vi "Plot menu activation.vi"(8 "error in (no error)":errorcluster, 11 "BluePlotHandle in":refnum<class "BluePlotHandle.lvclass">) -> (0 "error out":errorcluster, 2 "item tags":string[](array[string]), 3 "BluePlotHandle out":refnum<class "BluePlotHandle.lvclass">)   [LabVIEW 2021, in "BluePlot.lvlib" / "BluePlotHandle.lvclass"]
uses:
  BluePlotHandle.lvclass
  BluePlotHandle.lvclass/BluePlotHandle.ctl
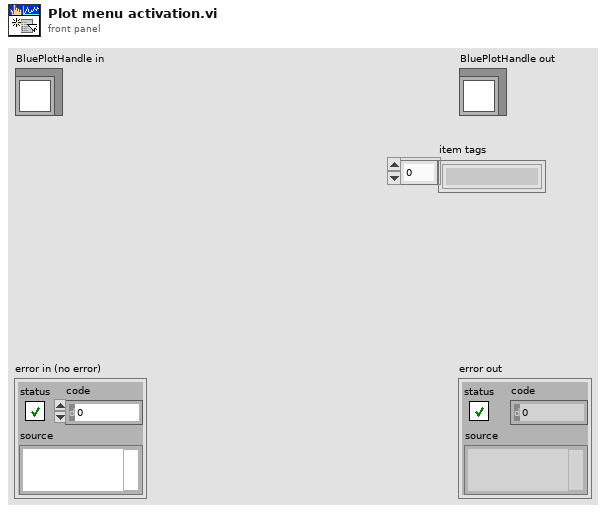
[diagram p1: front panel]
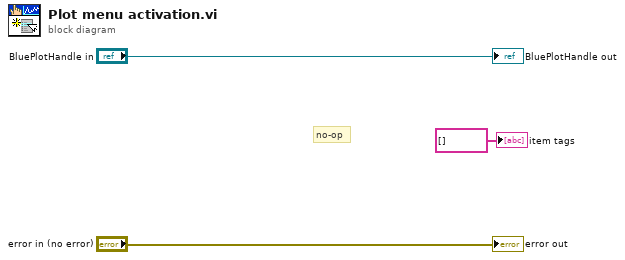
[diagram p0: block diagram]
diagram:
  # "no-op"
  "error out" <- "error in (no error)"
  "BluePlotHandle out" <- "BluePlotHandle in"
  "item tags" <- string[] [] ("item tags")
